vi "AlliGator Update Settings Guess Parameter Arrays.vi"(7 "Modified Control":string, 8 "Error In":errorcluster, 9 "Old Value":variant, 10 "Guess Parameter Names":refnum<vi>, 11 "Guess Parameters":refnum<vi>) -> (0 "Error Out":errorcluster, 2 "Guess Parameter Name Array":T1[](array[typedef]), 3 "Guess Parameter Array":dbl[](array[numeric]))   [LabVIEW 2021, in "AlliGator Settings.lvlib"]
doc: "Handles user modifications of the <B>Guess Parameter Names</b> and/or <B>Guess Parameter Values</B> in the Settings window. Ensures that both arrays have the same size."
uses:
  AlliGator Settings.lvlib
  Fits/IRF(X)PSED/Decay Fit Parameters In List.ctl
  781ec18c-9e5d-4a35-a130-22cd45fc26db.vi
  6c196a89-5246-4af8-8ae7-67091c27b178.vi
  ae48da77-102c-44f3-80a1-16f09820e3e2.vi
  b0ef72a0-cf76-4a7d-a487-2ad4d6a0e4f9.vi
  254ab70c-e628-45c4-b1b0-70d8101e2926.vi
  781ec18c-9e5d-4a35-a130-22cd45fc26db.vi/66edaa57-c3d2-4b95-9a59-34162fac150a.vi
  781ec18c-9e5d-4a35-a130-22cd45fc26db.vi/fc21e6f1-d027-477b-a5a8-3ddf091112fd.vi
  6c196a89-5246-4af8-8ae7-67091c27b178.vi/e3f056c9-b380-47c9-81df-cb9e668e7929.vi
  ae48da77-102c-44f3-80a1-16f09820e3e2.vi/66edaa57-c3d2-4b95-9a59-34162fac150a.vi
  ae48da77-102c-44f3-80a1-16f09820e3e2.vi/fc21e6f1-d027-477b-a5a8-3ddf091112fd.vi
  254ab70c-e628-45c4-b1b0-70d8101e2926.vi/e3f056c9-b380-47c9-81df-cb9e668e7929.vi
  <userlib>/_OpenG.lib/array/array.llb/Sort Array__ogtk.vi
  <userlib>/_OpenG.lib/array/array.llb/Sort 1D Array (I32)__ogtk.vi
  <userlib>/_OpenG.lib/array/array.llb/Reorder Array2__ogtk.vi
  <userlib>/_OpenG.lib/array/array.llb/Reorder 1D Array2 (I32)__ogtk.vi
  <userlib>/_OpenG.lib/array/array.llb/Delete Elements from 1D Array (DBL)__ogtk.vi
  <userlib>/_OpenG.lib/array/array.llb/Remove Duplicates from 1D Array (U16)__ogtk.vi
  <userlib>/_OpenG.lib/array/array.llb/openg_array.lvlib
  Fits/Fits.lvlib
panel:
  # "see the AlliGator License on the block diagram (Ctrl+E or Window:Show Block Diagram)"
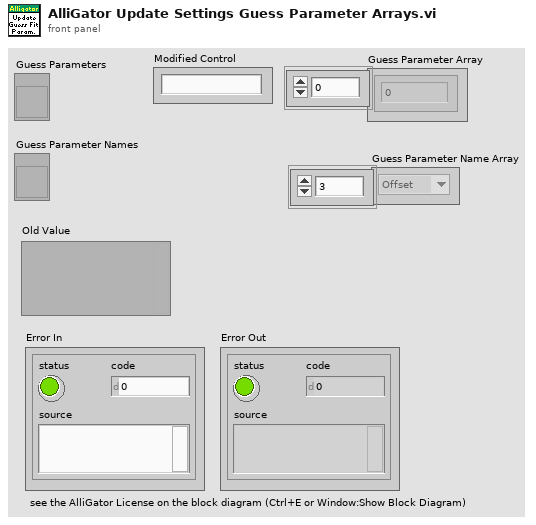
[diagram p1: front panel]
types:
  T1 = typedef "Fits.lvlib/Decay Fit Parameters In List.ctl" = enum16{"Offset", "Baseline", "A_1", "tau_1", "A_2", "tau_2"}
  T2 = typedef "Decay Fit Parameters In List.ctl" = enum16{"Offset", "Baseline", "A_1", "tau_1", "A_2", "tau_2"}
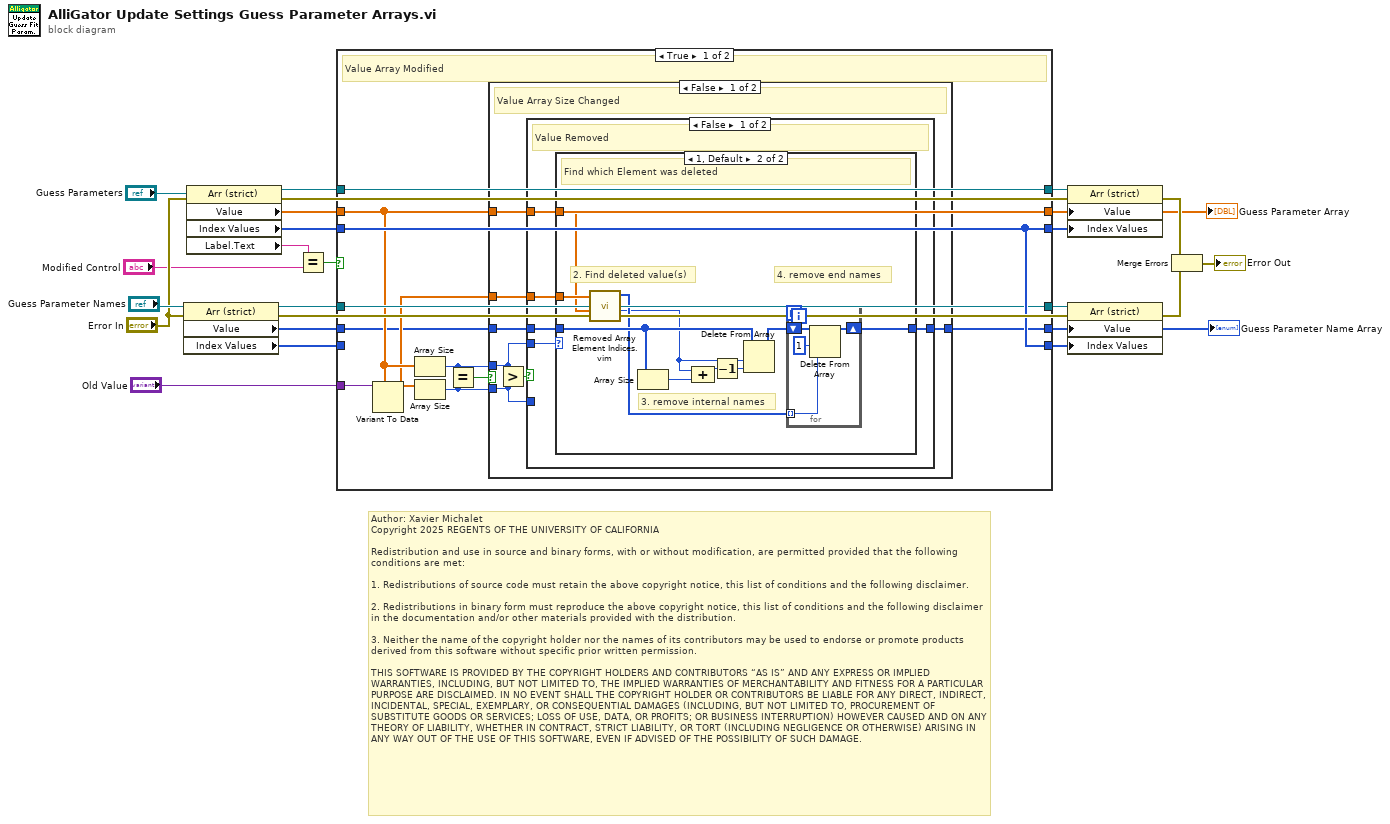
[diagram p0: block diagram]
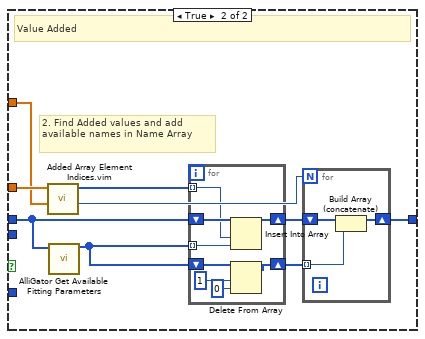
[diagram p3: hidden frame]
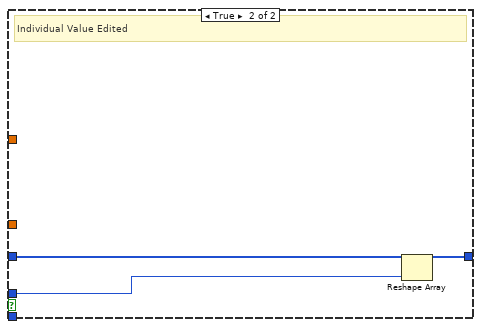
[diagram p4: hidden frame]
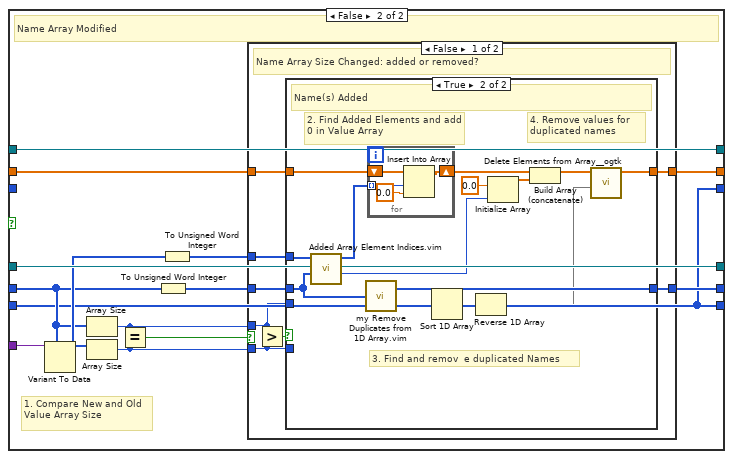
[diagram p5: hidden frame]
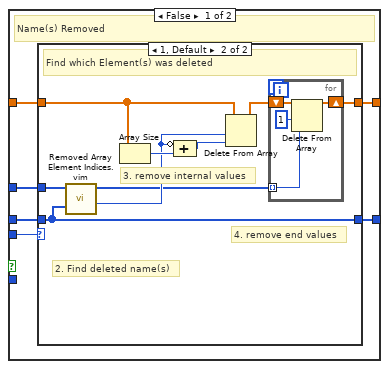
[diagram p6: hidden frame]
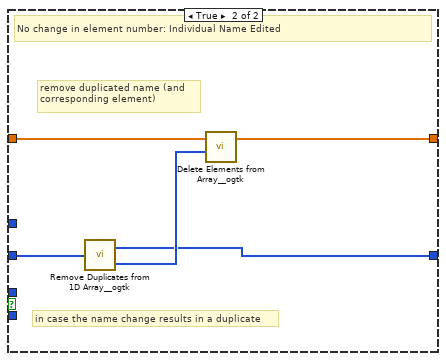
[diagram p8: hidden frame]
diagram:
  # "Author: Xavier Michalet\nCopyright 2025 REGENTS OF THE UNIVERSITY OF CALIFORNIA\n\nRedistribution and use in source and binary forms, with or without modification, are permitted provided that the following conditions are met:\n\n1. Redistributions of source code must retain the above copyright notice, this list of conditions and the following disclaimer.\n\n2. Redistributions in binary form must reproduce the above copyright notice, this list of conditions and the following disclaimer in the documentation and/or other materials provided with the distribution.\n\n3. Neither the name of the copyright holder nor the names of its contributors may be used to endorse or promote products derived from this software without specific prior written permission.\n\nTHIS SOFTWARE IS PROVIDED BY THE COPYRIGHT HOLDERS AND CONTRIBUTORS “AS IS” AND ANY EXPRESS OR IMPLIED WARRANTIES, INCLUDING, BUT NOT LIMITED TO, THE IMPLIED WARRANTIES OF MERCHANTABILITY AND FITNESS FOR A PARTICULAR PURPOSE ARE DISCLAIMED. IN NO EVENT SHALL THE COPYRIGHT HOLDER OR CONTRIBUTORS BE LIABLE FOR ANY DIRECT, INDIRECT, INCIDENTAL, SPECIAL, EXEMPLARY, OR CONSEQUENTIAL DAMAGES (INCLUDING, BUT NOT LIMITED TO, PROCUREMENT OF SUBSTITUTE GOODS OR SERVICES; LOSS OF USE, DATA, OR PROFITS; OR BUSINESS INTERRUPTION) HOWEVER CAUSED AND ON ANY THEORY OF LIABILITY, WHETHER IN CONTRACT, STRICT LIABILITY, OR TORT (INCLUDING NEGLIGENCE OR OTHERWISE) ARISING IN ANY WAY OUT OF THE USE OF THIS SOFTWARE, EVEN IF ADVISED OF THE POSSIBILITY OF SUCH DAMAGE."
  n1 = property class="Arr (strict)"(reference="Guess Parameter Names", error in="Error In") -> (reference out=w12:refnum<vi>, error out=w9:errorcluster, "Value"=w14:T2[], "Index Values"=w13:u32[])
  n2 = property class="Arr (strict)"(reference="Guess Parameters", error in="Error In") -> (reference out=w17:refnum<vi>, error out=w6:errorcluster, "Value"=w20:dbl[], "Index Values"=w19:u32[], "Label.Text"=w7:string)
  n3 = Equal?(x=w7, y="Modified Control") -> (x = y?=w22:bool)
  n4 = case shown="True" w22 {
    tunnel: "Old Value" -> [w35 w98]
    tunnel: w20 -> [w28 w92]
    tunnel: w19 -> [w33 _]
    tunnel: [w33 w87] -> w18
    tunnel: [w28 w88] -> w2
    tunnel: w17 -> [w34 w97]
    tunnel: [w34 w97] -> w16
    tunnel: [w33 w87] -> w15
    tunnel: w14 -> [w26 w89]
    tunnel: w13 -> [_ w87]
    tunnel: [w25 w90] -> w1
    tunnel: w12 -> [w32 w96]
    tunnel: [w32 w96] -> w11
    frame True {
      # "Value Array Modified"
      n5 = Variant To Data(type=w28, Variant=w35) -> (data=w27:dbl[])  [unwired: 1 in, 1 out]
      n6 = Array Size(array=w28) -> (size(s)=w30:i32)
      n7 = Array Size(array=w27) -> (size(s)=w29:i32)
      n8 = Equal?(x=w30, y=w29) -> (x = y?=w31:bool)
      n9 = case shown="False" w31 {
        tunnel: w30 -> [w37 w82]
        tunnel: w29 -> [w36 _]
        tunnel: w28 -> [w41 _]
        tunnel: w27 -> [w40 _]
        tunnel: w26 -> [w39 w84]
        tunnel: [w38 w83] -> w25
        frame False {
          # "Value Array Size Changed"
          n10 = Greater?(x=w37, y=w36) -> (0:w42:bool)
          n11 = case shown="False" w42 {
            tunnel: w41 -> [w46 w63]
            tunnel: w40 -> [w45 w70]
            tunnel: w39 -> [w44 w68]
            tunnel: [w43 w65] -> w38
            tunnel: w37 -> [w47 _]
            tunnel: w36 -> [_ _]
            frame False {
              # "Value Removed"
              n12 = case shown="1, Default" w47 {
                tunnel: w46 -> [_ w56]
                tunnel: w45 -> [_ w57]
                tunnel: w44 -> [_ w51]
                tunnel: [_ w48] -> w43
                frame 0 {
                  # "No element left"
                }
                frame 1, Default {
                  # "4. remove end names"
                  # "2. Find deleted value(s)"
                  # "3. remove internal names"
                  # "Find which Element was deleted"
                  n13 = call "Removed Array Element Indices.vim"("New Array"=w56, "Old Array"=w57) -> ("# End Elements Deleted"=w49:i32, "Removed Element Indices (Internal, \\ order)"=w50:i32[])  [unwired: 8 in]
                  n14 = Array Size(array=w51) -> (size(s)=w55:i32)
                  n15 = Compound Arithmetic op=ADD(w49, w55) -> (w54:i32)
                  n16 = Decrement(x=w54) -> (x-1=w53:i32)
                  n17 = Delete From Array(array=w51, length=w49, index=w53) -> (array with subset deleted=w52:T2[])  [unwired: 1 out]
                  n18 = for {
                    shift-right: [w59] -> w48
                    shift-left: w52 -> [w60]
                    tunnel: w50 -> [w58] mode=indexing
                    n19 = Delete From Array(array=w60, length=1, index=w58) -> (array with subset deleted=w59:T2[])  [unwired: 1 out]
                  }
                }
              }
            }
            frame True {
              # "2. Find Added values and add available names in Name Array"
              # "Value Added"
              n20 = call "Added Array Element Indices.vim"("New Array"=w63, "Old Array"=w70) -> ("# Appended Elements"=w62:i32, "Inserted Element Indices in Old Array (\\ order)"=w69:i32[])  [unwired: 6 in, 2 out]
              n21 = call "AlliGator Get Available Fitting Parameters.vi"("Parameter Names"=w68) -> ("Missing Parameter Names"=w67:T1[])  [unwired: 10 in]
              n22 = for {
                tunnel: w69 -> [w80] mode=indexing
                shift-right: [w78] -> w66
                shift-left: w68 -> [w81]
                tunnel: w67 -> [w79] mode=indexing
                shift-right: [w74] -> w64
                shift-left: w67 -> [w77]
                n23 = Insert Into Array(array=w81, index=w80, new element=w79) -> (w78:T2[])
                n24 = Delete From Array(array=w77, length=1, index=0) -> (array with subset deleted=w74:T1[])  [unwired: 1 out]
              }
              n25 = for {
                N: w62 -> [_]
                shift-right: [w71] -> w65
                shift-left: w66 -> [w73]
                tunnel: w64 -> [w72] mode=indexing
                n26 = Build Array (concatenate)(w73, w72) -> (w71:T1[])
              }
            }
          }
        }
        frame True {
          # "Individual Value Edited"
          n27 = Reshape Array(w84, w82) -> (w83:T2[])
        }
      }
    }
    frame False {
      # "1. Compare New and Old Value Array Size"
      # "Name Array Modified"
      n28 = Variant To Data(type=w89, Variant=w98) -> (data=w91:T2[])  [unwired: 1 in, 1 out]
      n29 = Array Size(array=w89) -> (size(s)=w94:i32)
      n30 = Array Size(array=w91) -> (size(s)=w93:i32)
      n31 = Equal?(x=w94, y=w93) -> (x = y?=w95:bool)
      n32 = To Unsigned Word Integer(number=w89) -> (unsigned 16bit integer=w86:u16[])
      n33 = To Unsigned Word Integer(number=w91) -> (unsigned 16bit integer=w85:u16[])
      n34 = case shown="False" w95 {
        tunnel: w94 -> [w101 _]
        tunnel: w93 -> [w99 _]
        tunnel: w92 -> [w105 w146]
        tunnel: w85 -> [w104 _]
        tunnel: w86 -> [w103 w144]
        tunnel: [w102 w145] -> w90
        tunnel: [w100 w146] -> w88
        frame False {
          # "Name Array Size Changed: added or removed?"
          n35 = Greater?(x=w101, y=w99) -> (0:w106:bool)
          n36 = case shown="True" w106 {
            tunnel: w105 -> [w111 w138]
            tunnel: w104 -> [w110 w139]
            tunnel: w103 -> [w109 w126]
            tunnel: [w108 w131] -> w102
            tunnel: w101 -> [w112 _]
            tunnel: [w107 w127] -> w100
            tunnel: w99 -> [_ _]
            frame False {
              # "Name(s) Removed"
              n37 = case shown="1, Default" w112 {
                tunnel: w111 -> [_ w115]
                tunnel: w110 -> [_ w121]
                tunnel: w109 -> [_ w119]
                tunnel: [_ w119] -> w108
                tunnel: [_ w120] -> w107
                frame 0 {
                  # "empty value array"
                  # "No element left"
                }
                frame 1, Default {
                  # "4. remove end values"
                  # "3. remove internal values"
                  # "2. Find deleted name(s)"
                  # "Find which Element(s) was deleted"
                  n38 = call "Removed Array Element Indices.vim"("New Array"=w119, "Old Array"=w121) -> ("# End Elements Deleted"=w117:i32, "Removed Element Indices (Internal, \\ order)"=w114:i32[])  [unwired: 8 in]
                  n39 = Array Size(array=w115) -> (size(s)=w118:i32)
                  n40 = Compound Arithmetic op=ADD(invert w117, w118) -> (w113:i32)
                  n41 = Delete From Array(array=w115, length=w117, index=w113) -> (array with subset deleted=w116:dbl[])  [unwired: 1 out]
                  n42 = for {
                    shift-right: [w123] -> w120
                    shift-left: w116 -> [w124]
                    tunnel: w114 -> [w122] mode=indexing
                    n43 = Delete From Array(array=w124, length=1, index=w122) -> (array with subset deleted=w123:dbl[])  [unwired: 1 out]
                  }
                }
              }
            }
            frame True {
              # "4. Remove values for duplicated names"
              # "3. Find and remov  e duplicated Names"
              # "2. Find Added Elements and add 0 in Value Array"
              # "Name(s) Added"
              n44 = call "Added Array Element Indices.vim"("New Array"=w126, "Old Array"=w139) -> ("# Appended Elements"=w134:i32, "Inserted Element Indices in Old Array (\\ order)"=w136:i32[])  [unwired: 6 in, 2 out]
              n45 = call "my Remove Duplicates from 1D Array.vim"("Input Array"=w126) -> ("Output Array"=w131:u16[], "indices of removed elements"=w130:i32[])
              n46 = for {
                shift-right: [w140] -> w137
                shift-left: w138 -> [w143]
                tunnel: w136 -> [w142] mode=indexing
                n47 = Insert Into Array(array=w143, index=w142, new element=0.0 ("new element/subarray")) -> (w140:dbl[])
              }
              n48 = Sort 1D Array(array=w130) -> (sorted array=w129:i32[])
              n49 = Reverse 1D Array(array=w129) -> (reversed array=w128:i32[])
              n50 = Initialize Array(0.0 ("element"), w134) -> (w133:dbl[])
              n51 = Build Array (concatenate)(w137, w133) -> (w135:dbl[])
              n52 = call-poly <userlib>:"Delete Elements from Array__ogtk.vi"("indices"=w128, "array"=w135) -> ("array w/ subset deleted"=w127:dbl[])  [unwired: 8 in, 1 out]
            }
          }
        }
        frame True {
          # "remove duplicated name (and corresponding element)"
          # "in case the name change results in a duplicate"
          # "No change in element number: Individual Name Edited"
          n53 = call-poly <userlib>:"Remove Duplicates from 1D Array__ogtk.vi"("Input Array"=w144) -> ("Output Array"=w145:u16[], "indices of removed elements"=w147:i32[])
          n54 = call-poly <userlib>:"Delete Elements from Array__ogtk.vi"("indices"=w147, "array"=w146) -> ()  [unwired: 8 in, 2 out]
        }
      }
    }
  }
  "Guess Parameter Array" <- w2
  "Guess Parameter Name Array" <- w1
  n55 = property class="Arr (strict)"(reference=w16, error in=w6, "Value"=w2, "Index Values"=w18) -> (error out=w5:errorcluster)  [unwired: 1 out]
  n56 = property class="Arr (strict)"(reference=w11, error in=w9, "Value"=w1, "Index Values"=w15) -> (error out=w4:errorcluster)  [unwired: 1 out]
  n57 = Merge Errors(w5, w4) -> (→"Error Out":errorcluster)
